vi "Helper-WaypointToRelative.vi"(9 "Next Waypoint":refnum<class "Waypoint.lvclass">, 10 "Boat location":T1 {"North" format="%#_10f"; "East" format="%#_8f"}) -> (2 "Relative Waypoint":cluster{"X":dbl, "Y":dbl})   [LabVIEW 2013]
doc: "Translates the next waypoint into coordinates relative to the current boat (that is, transform it such that current boat location is (0,0)). This makes the tacking math easier.\n\n-Elizabeth Mahon, 12/20/2014"
uses:
  Data/TypeDefs/UTM Location.ctl
  Classes/Waypoint/Waypoint.lvclass
panel:
  in  "Coords (for testing)":T1 {"North" format="%#_10f"; "East" format="%#_8f"}
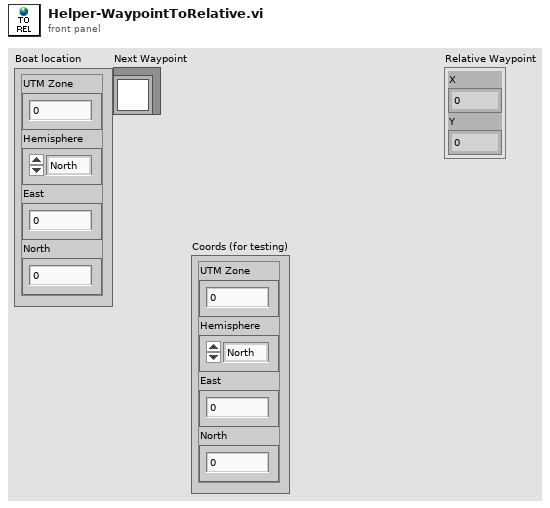
[diagram p1: front panel]
types:
  T1 = typedef "UTM Location.ctl" = cluster{"UTM Zone":dbl, "Hemisphere":enum16{"North", "South"}, "East":dbl, "North":dbl}
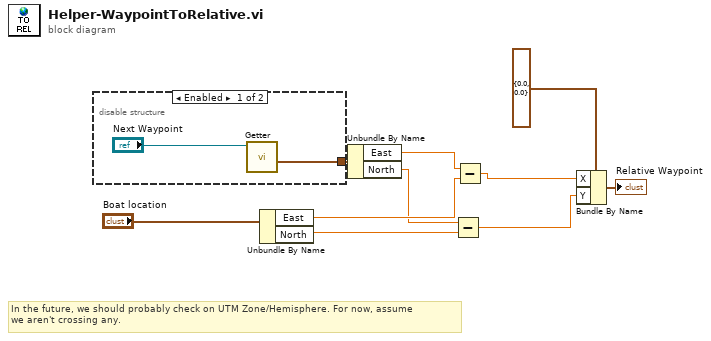
[diagram p0: block diagram]
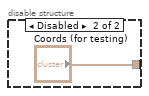
[diagram p2: hidden frame]
diagram:
  # "In the future, we should probably check on UTM Zone/Hemisphere. For now, assume\nwe aren't crossing any."
  n1 = disable-structure shown="Enabled" {
    disable-tunnel: [w11 "Coords (for testing)"] -> w9
    frame Enabled {
      n2 = call "Getter.vi"("Waypoint In"="Next Waypoint") -> ("Coords"=w11:T1)  [unwired: 5 in, 5 out]
    }
    frame Disabled {
    }
  }
  n3 = Unbundle By Name("Boat location") -> ("East"=w7:dbl, "North"=w5:dbl)
  n4 = Unbundle By Name(w9) -> ("East"=w8:dbl, "North"=w6:dbl)
  n5 = Subtract(x=w6, y=w5) -> (x-y=w2:dbl)
  n6 = Subtract(x=w8, y=w7) -> (x-y=w3:dbl)
  n7 = Bundle By Name(cluster=cluster{"X":dbl, "Y":dbl} {"X"=0.0, "Y"=0.0} ("input cluster"), "X"=w3, "Y"=w2) -> (→"Relative Waypoint":cluster{"X":dbl, "Y":dbl})
